vi "Send Message.vi"(8 "error in":errorcluster, 9 "Value":dbl, 10 "Message to Send":T1, 11 "EF20 in":refnum<class "EF20.lvclass">) -> (0 "error out":errorcluster, 3 "EF20 out":refnum<class "EF20.lvclass">)   [LabVIEW 2018, in "EF20.lvlib" / "EF20.lvclass"]
uses:
  EF20.lvclass
  PPLs/Oven/Oven.lvlibp/Custom Controls/Message Type.ctl
  Custom Controls/EF20 Message Type.ctl
  EF20.lvclass/EF20.ctl
  EF20.lvlib
  PPLs/Oven/Oven.lvlibp/Oven.lvclass
  C:/Projects/LabVIEW/PPLs/Oven/Oven.lvlibp/Oven.lvclass
  PPLs/Oven/Oven.lvlibp
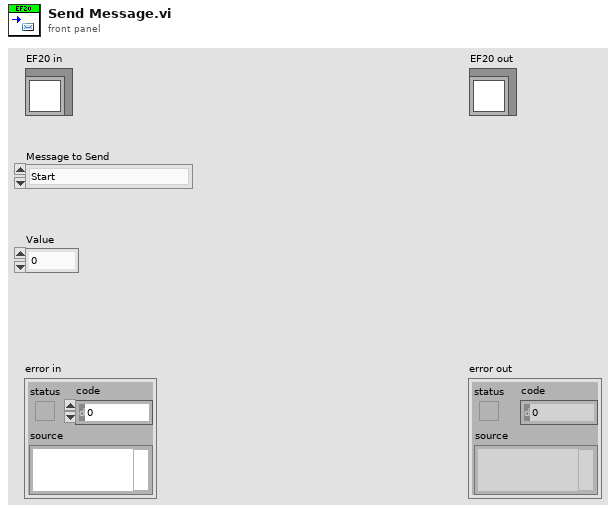
[diagram p1: front panel]
types:
  T1 = typedef "Oven.lvlibp/Message Type.ctl" = enum16{"Start", "Stop", "Set Temperature", "Get Temperature"}
  T2 = typedef "EF20.lvlib/EF20 Message Type.ctl" = u8
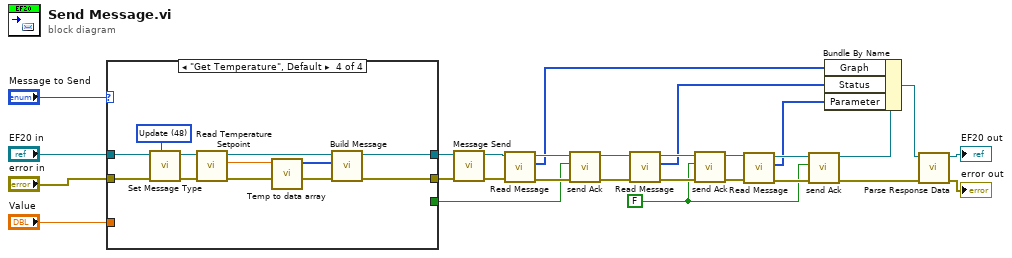
[diagram p0: block diagram]
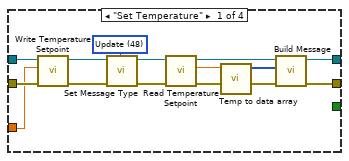
[diagram p2: hidden frame]
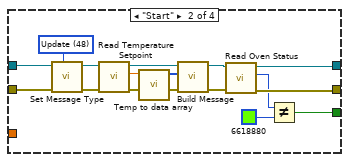
[diagram p3: hidden frame]
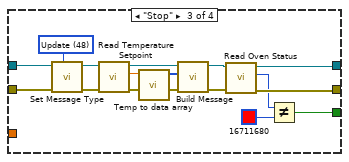
[diagram p4: hidden frame]
diagram:
  w5 = FALSE
  n1 = case shown="\"Get Temperature\", Default" "Message to Send" {
    tunnel: "EF20 in" -> [w39 w58 w74 w85]
    tunnel: [w42 w47 w63 w83] -> w23
    tunnel: "Value" -> [w34 _ _ _]
    tunnel: "error in" -> [w38 w57 w73 w84]
    tunnel: [w41 w46 w62 w82] -> w24
    tunnel: [_ w43 w59 _] -> w6
    frame "Set Temperature" {
      w40 = T2 48 items=["Update"=48, "Graph"=49, "Status"=50, "Parameter"=51, "Acknowledge"=1] ("EF20 Message type")
      n2 = call "Write Temperature Setpoint.vi"("error in (no error)"=w38, "Temperature Setpoint"=w34, "Oven in"=w39) -> ("error out"=w36:errorcluster, "Oven out"=w37:refnum<class "EF20.lvclass">)  [unwired: 7 in]
      n3 = call "Set Message Type.vi"("EF20 Message type"=w40, "error in"=w36, "EF20 in"=w37) -> ("error out"=w33:errorcluster, "EF20 out"=w32:refnum<class "EF20.lvclass">)  [unwired: 7 in]
      n4 = call "Read Temperature Setpoint.vi"("error in (no error)"=w33, "Oven in"=w32) -> ("error out"=w30:errorcluster, "Temperature Setpoint"=w29:dbl, "Oven out"=w31:refnum<class "EF20.lvclass">)  [unwired: 7 in]
      n5 = call "Temp to data array.vi"("Temperature"=w29) -> ("Data"=w35:u8[])  [unwired: 10 in]
      n6 = call "Build Message.vi"("error in (no error)"=w30, "Data to Send"=w35, "EF20 in"=w31) -> ("error out"=w41:errorcluster, "EF20 out"=w42:refnum<class "EF20.lvclass">)  [unwired: 7 in]
    }
    frame "Start" {
      w56 = T2 48 items=["Update"=48, "Graph"=49, "Status"=50, "Parameter"=51, "Acknowledge"=1] ("EF20 Message type")
      n7 = call "Set Message Type.vi"("EF20 Message type"=w56, "error in"=w57, "EF20 in"=w58) -> ("error out"=w54:errorcluster, "EF20 out"=w53:refnum<class "EF20.lvclass">)  [unwired: 7 in]
      n8 = call "Read Temperature Setpoint.vi"("error in (no error)"=w54, "Oven in"=w53) -> ("error out"=w55:errorcluster, "Temperature Setpoint"=w51:dbl, "Oven out"=w52:refnum<class "EF20.lvclass">)  [unwired: 7 in]
      n9 = call "Temp to data array.vi"("Temperature"=w51) -> ("Data"=w50:u8[])  [unwired: 10 in]
      n10 = call "Build Message.vi"("error in (no error)"=w55, "Data to Send"=w50, "EF20 in"=w52) -> ("error out"=w49:errorcluster, "EF20 out"=w48:refnum<class "EF20.lvclass">)  [unwired: 7 in]
      n11 = call "Read Oven Status.vi"("error in (no error)"=w49, "Oven in"=w48) -> ("error out"=w46:errorcluster, "Oven Status"=w45:u32, "Oven out"=w47:refnum<class "EF20.lvclass">)  [unwired: 7 in]
      n12 = Not Equal?(x=w45, y=u32 6618880 ("Oven Status")) -> (x != y?=w43:bool)
    }
    frame "Stop" {
      w72 = T2 48 items=["Update"=48, "Graph"=49, "Status"=50, "Parameter"=51, "Acknowledge"=1] ("EF20 Message type")
      n13 = call "Set Message Type.vi"("EF20 Message type"=w72, "error in"=w73, "EF20 in"=w74) -> ("error out"=w70:errorcluster, "EF20 out"=w69:refnum<class "EF20.lvclass">)  [unwired: 7 in]
      n14 = call "Read Temperature Setpoint.vi"("error in (no error)"=w70, "Oven in"=w69) -> ("error out"=w71:errorcluster, "Temperature Setpoint"=w67:dbl, "Oven out"=w68:refnum<class "EF20.lvclass">)  [unwired: 7 in]
      n15 = call "Temp to data array.vi"("Temperature"=w67) -> ("Data"=w66:u8[])  [unwired: 10 in]
      n16 = call "Build Message.vi"("error in (no error)"=w71, "Data to Send"=w66, "EF20 in"=w68) -> ("error out"=w65:errorcluster, "EF20 out"=w64:refnum<class "EF20.lvclass">)  [unwired: 7 in]
      n17 = call "Read Oven Status.vi"("error in (no error)"=w65, "Oven in"=w64) -> ("error out"=w62:errorcluster, "Oven Status"=w61:u32, "Oven out"=w63:refnum<class "EF20.lvclass">)  [unwired: 7 in]
      n18 = Not Equal?(x=w61, y=u32 16711680 ("Oven Status")) -> (x != y?=w59:bool)
    }
    frame "Get Temperature", Default {
      w81 = T2 48 items=["Update"=48, "Graph"=49, "Status"=50, "Parameter"=51, "Acknowledge"=1] ("EF20 Message type")
      n19 = call "Set Message Type.vi"("EF20 Message type"=w81, "error in"=w84, "EF20 in"=w85) -> ("error out"=w79:errorcluster, "EF20 out"=w78:refnum<class "EF20.lvclass">)  [unwired: 7 in]
      n20 = call "Read Temperature Setpoint.vi"("error in (no error)"=w79, "Oven in"=w78) -> ("error out"=w80:errorcluster, "Temperature Setpoint"=w76:dbl, "Oven out"=w77:refnum<class "EF20.lvclass">)  [unwired: 7 in]
      n21 = call "Temp to data array.vi"("Temperature"=w76) -> ("Data"=w75:u8[])  [unwired: 10 in]
      n22 = call "Build Message.vi"("error in (no error)"=w80, "Data to Send"=w75, "EF20 in"=w77) -> ("error out"=w82:errorcluster, "EF20 out"=w83:refnum<class "EF20.lvclass">)  [unwired: 7 in]
    }
  }
  n23 = call "Message Send.vi"("error in"=w24, "EF20 in"=w23) -> ("error out"=w21:errorcluster, "EF20 out"=w22:refnum<class "EF20.lvclass">)  [unwired: 8 in]
  n24 = call-dynamic "Read Message.vi"("error in"=w21, "EF20 in"=w22) -> ("error out"=w19:errorcluster, "Read Data"=w9:u8[], "EF20 out"=w20:refnum<class "EF20.lvclass">)  [unwired: 7 in]
  n25 = call "send Ack.vi"("error in"=w19, "State Change?"=w6, "EF20 in"=w20) -> ("error out"=w18:errorcluster, "EF20 out"=w17:refnum<class "EF20.lvclass">)  [unwired: 7 in]
  n26 = call-dynamic "Read Message.vi"("error in"=w18, "EF20 in"=w17) -> ("error out"=w15:errorcluster, "Read Data"=w8:u8[], "EF20 out"=w16:refnum<class "EF20.lvclass">)  [unwired: 7 in]
  n27 = call "send Ack.vi"("error in"=w15, "State Change?"=w5, "EF20 in"=w16) -> ("error out"=w12:errorcluster, "EF20 out"=w11:refnum<class "EF20.lvclass">)  [unwired: 7 in]
  n28 = call-dynamic "Read Message.vi"("error in"=w12, "EF20 in"=w11) -> ("error out"=w14:errorcluster, "Read Data"=w7:u8[], "EF20 out"=w13:refnum<class "EF20.lvclass">)  [unwired: 7 in]
  n29 = call "send Ack.vi"("error in"=w14, "State Change?"=w5, "EF20 in"=w13) -> ("error out"=w2:errorcluster, "EF20 out"=w10:refnum<class "EF20.lvclass">)  [unwired: 7 in]
  n30 = Bundle By Name(cluster=w10, "Graph"=w9, "Status"=w8, "Parameter"=w7) -> (w3:refnum<class "EF20.lvclass">)
  n31 = call "Parse Response Data.vi"("error in"=w2, "EF20 in"=w3) -> ("error out"=→"error out":errorcluster, "EF20 out"=→"EF20 out":refnum<class "EF20.lvclass">)  [unwired: 8 in]
